vi "Save strain data.vi"(8 "Error In":errorcluster, 10 "Data":dbl[][](array[numeric])) -> (0 "Error Out":errorcluster, 3 "File name":path)   [LabVIEW 2015]
uses:
  File/Controls/File formats.ctl
  <vilib>/Utility/file.llb/Write To Spreadsheet File (DBL).vi
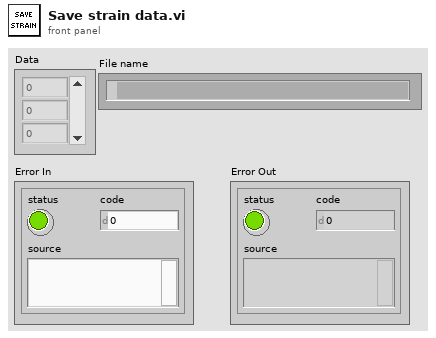
[diagram p1: front panel]
types:
  T1 = typedef "File formats.ctl" = enum16{"TDMS", "ASCII", "BINARY"}
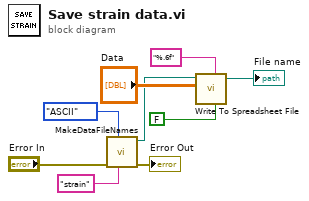
[diagram p0: block diagram]
diagram:
  n1 = call "MakeDataFileNames.vi"("File Prefix"="strain" ("File Name Prefix"), "File format"=File_formats."ASCII", "Error In"="Error In") -> ("Error Out"=→"Error Out":errorcluster, "Data File  Path"=w4:path)  [unwired: 5 in, 2 out]
  n2 = call-poly <vilib>:"Write To Spreadsheet File.vi"("transpose? (no:F)"=FALSE, "format (%.3f)"="%.6f", "2D data"="Data", "file path (dialog if empty)"=w4) -> ("new file path (Not A Path if cancelled)"=→"File name":path)  [unwired: 4 in]
